vi "Write stop.vi"(8 "error in (no error)":errorcluster, 10 "Stop":bool, 11 "MB in":refnum<class "Modbus Master CR.lvclass">) -> (0 "error out":errorcluster, 3 "MB out":refnum<class "Modbus Master CR.lvclass">)   [LabVIEW 2021, in "Modbus Master CR.lvclass"]
uses:
  Modbus Master CR.lvclass
  Modbus Master CR.lvclass/Modbus Master CR.ctl
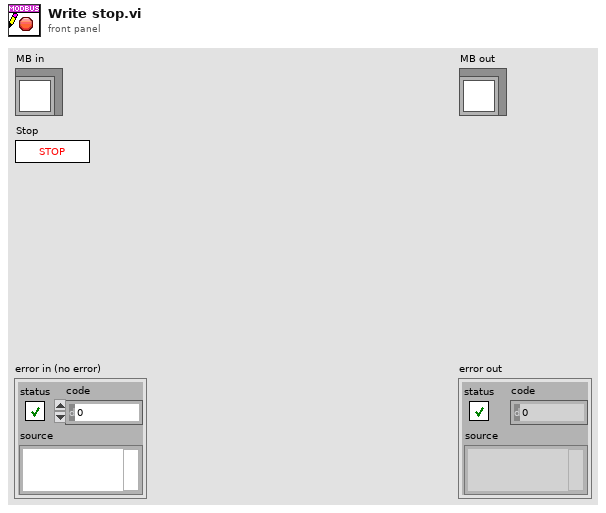
[diagram p1: front panel]
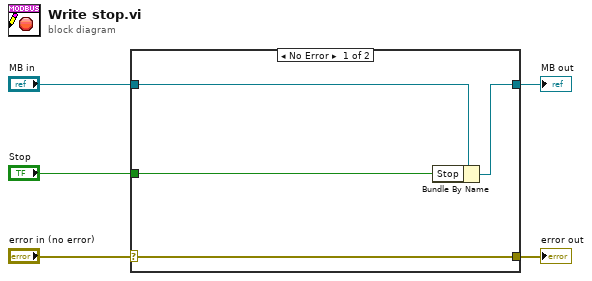
[diagram p0: block diagram]
diagram:
  n1 = case shown="No Error" "error in (no error)" {
    selector: "error in (no error)" -> [w9 w10]
    tunnel: [w9 w10] -> w4
    tunnel: [w7 w11] -> w2
    tunnel: "MB in" -> [w8 w11]
    tunnel: "Stop" -> [w6 _]
    frame No Error {
      n2 = Bundle By Name(cluster=w8, "Stop"=w6) -> (w7:refnum<class "Modbus Master CR.lvclass">)
    }
    frame Error {
    }
  }
  "error out" <- w4
  "MB out" <- w2
